vi "Make K-Points File, Auto.vi"(6 "|G| Factor":dbl=30.0, 8 "Lattice vector c":dbl[](array[numeric]), 9 "Lattice vector b":dbl[](array[numeric]), 10 "Lattice vector a":dbl[](array[numeric]), 11 "Auto Type":T1(radio)) -> (3 "K-Points File":string="Automatic Mesh\n-1\nGamma Centered Monkhurst-Pack\n  NaN NaN NaN\n")   [LabVIEW 2010]
uses:
  <vilib>/Analysis/_algsub.llb/Real Vector Norm.vi
  <vilib>/Analysis/NI_AALPro.lvlib
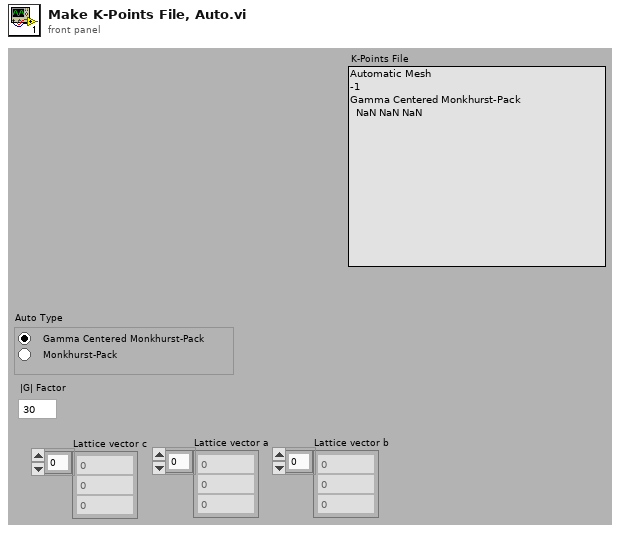
[diagram p1: front panel]
types:
  T1 = enum32{"Gamma Centered Monkhurst-Pack", "Monkhurst-Pack"}
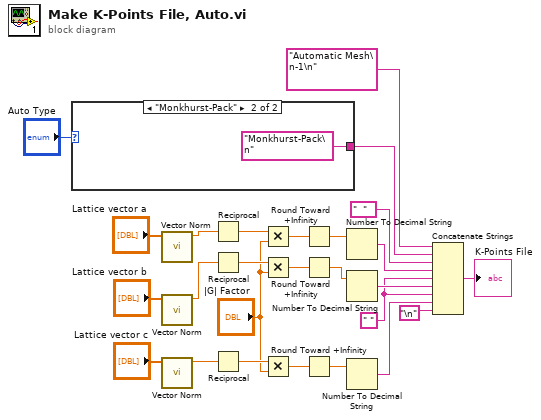
[diagram p0: block diagram]
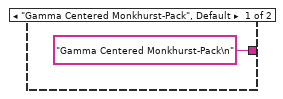
[diagram p2: hidden frame]
diagram:
  w9 = " " ("string")
  n1 = case shown="\"Monkhurst-Pack\"" "Auto Type" {
    tunnel: ["Gamma Centered Monkhurst-Pack\n" "Monkhurst-Pack\n"] -> w5
    frame "Gamma Centered Monkhurst-Pack", Default {
    }
    frame "Monkhurst-Pack" {
    }
  }
  n2 = call-poly <vilib>:"Vector Norm.vi"("Input Vector"="Lattice vector a") -> ("norm"=w23:dbl)  [unwired: 9 in, 1 out]
  n3 = call-poly <vilib>:"Vector Norm.vi"("Input Vector"="Lattice vector b") -> ("norm"=w20:dbl)  [unwired: 9 in, 1 out]
  n4 = call-poly <vilib>:"Vector Norm.vi"("Input Vector"="Lattice vector c") -> ("norm"=w17:dbl)  [unwired: 9 in, 1 out]
  n5 = Reciprocal(x=w23) -> (1/x=w24:dbl)
  n6 = Reciprocal(x=w20) -> (1/x=w19:dbl)
  n7 = Reciprocal(x=w17) -> (1/x=w18:dbl)
  n8 = Multiply(x=w24, y="|G| Factor") -> (x*y=w22:dbl)
  n9 = Multiply(x=w19, y="|G| Factor") -> (x*y=w21:dbl)
  n10 = Multiply(x=w18, y="|G| Factor") -> (x*y=w16:dbl)
  n11 = Round Toward +Infinity(x=w22) -> (ceil(x): smallest int >= x=w15:dbl)
  n12 = Round Toward +Infinity(x=w21) -> (ceil(x): smallest int >= x=w14:dbl)
  n13 = Round Toward +Infinity(x=w16) -> (ceil(x): smallest int >= x=w13:dbl)
  n14 = Number To Decimal String(number=w15) -> (decimal integer string=w11:string)  [unwired: 1 in]
  n15 = Number To Decimal String(number=w14) -> (decimal integer string=w10:string)  [unwired: 1 in]
  n16 = Number To Decimal String(number=w13) -> (decimal integer string=w8:string)  [unwired: 1 in]
  n17 = Concatenate Strings("Automatic Mesh\n-1\n", w5, "  " ("string"), w11, w9, w10, w9, w8, "\n") -> (→"K-Points File":string)
